vi "Testbench for 2 Smooth Controls.vi"() -> ()   [LabVIEW 2011]
doc: "sends square waves in to Rudder Angle and Sail Position to test Smoothed Setpoints.vi. User can view the smoothed output."
uses:
  2 Typedefs/setpoints to boat.ctl
  2 Typedefs/sail setpt.ctl
  2 Typedefs/rudder angle.ctl
  <vilib>/ptbypt/NI_PtbyPt.lvlib
panel:
  in  "frequency to sails":dbl=0.2 format="%0.4f"
  in  "stop":bool
  in  "Loop Delay (ms)":u32=10
  out "Setpoints in to 2 Smooth Setpoints.vi":T1
  in  "amplitude in to sails":dbl=1.0 format="%0.2f"
  out "Smoothed Setpoints out":T1
  in  "frequency to rudder":dbl=0.2 format="%0.4f"
  in  "Amplitude to rudder":dbl=50.0 format="%0.2f"
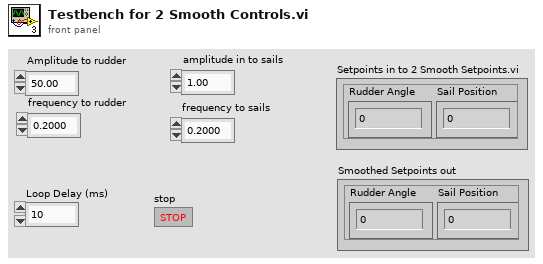
[diagram p1: front panel]
types:
  T1 = typedef "setpoints to boat.ctl" = cluster{"Sail Position":T2, "Rudder Angle":T3}
  T2 = typedef "sail setpt.ctl" = dbl
  T3 = typedef "rudder angle.ctl" = dbl
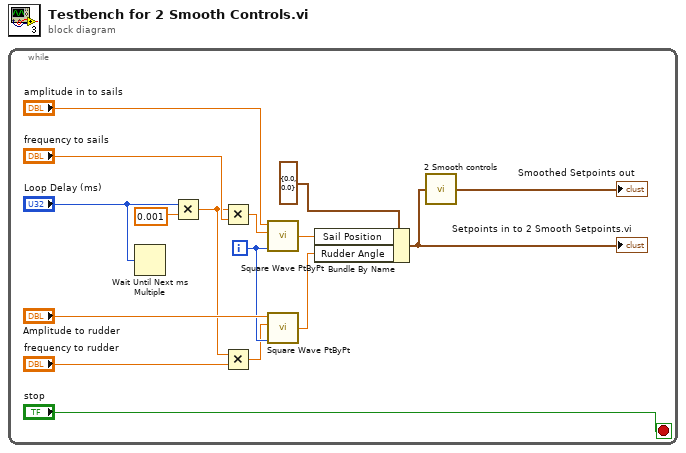
[diagram p0: block diagram]
diagram:
  n1 = while {
    i -> [w7]
    stop <- "stop" stop-if-true
    n2 = Wait Until Next ms Multiple(millisecond multiple="Loop Delay (ms)") -> ()  [unwired: 1 out]
    n3 = Multiply(x="Loop Delay (ms)", y=0.001 ("frequency to rudder 2")) -> (x*y=w1:dbl)
    n4 = Multiply(x=w1, y="frequency to sails") -> (x*y=w2:dbl)
    n5 = Multiply(x=w1, y="frequency to rudder") -> (x*y=w3:dbl)
    n6 = call <vilib>:"Square Wave PtByPt.vi"("amplitude"="amplitude in to sails", "frequency"=w2, "time"=w7) -> ("square wave"=w9:dbl)  [unwired: 2 in]
    n7 = call <vilib>:"Square Wave PtByPt.vi"("amplitude"="Amplitude to rudder", "frequency"=w3, "time"=w7) -> ("square wave"=w14:dbl)  [unwired: 2 in]
    n8 = Bundle By Name(cluster=T1 {"Sail Position"=0.0, "Rudder Angle"=0.0} ("Smoothed Setpoints out"), "Sail Position"=w9, "Rudder Angle"=w14) -> (w16:T1)
    "Setpoints in to 2 Smooth Setpoints.vi" <- w16
    n9 = call "2 Smooth controls.vi"("Setpoints in"=w16) -> ("Smoothed Setpoints out"=→"Smoothed Setpoints out":T1)  [unwired: 4 in]
  }
